vi "Prueba 2 Tania.vi"() -> ()   [LabVIEW 2013]
panel:
  out "mayor":dbl
  out "Menor":dbl
  out "Temperatura80":dbl
  out "Promedio":dbl
  out "Velocidad":i32(knob) scale=0.0..220.0
  # "Necesitamos generar 10 velocidades. \nal final de las 10 pruebas presentar :\n-Promedio de las velocidades mayores a 120\n-Velocidad Mayor y menor \n-Cuantas veces la temperatura fue mayor a 80"
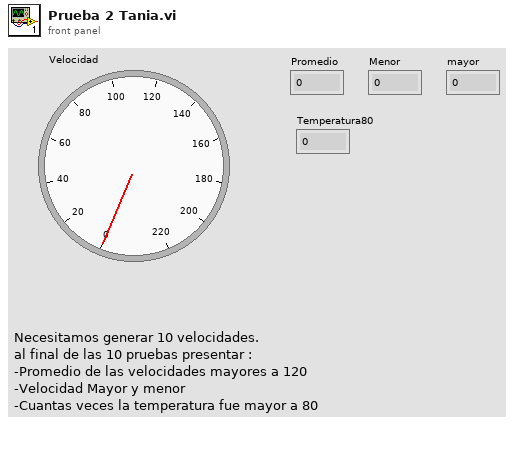
[diagram p1: front panel]
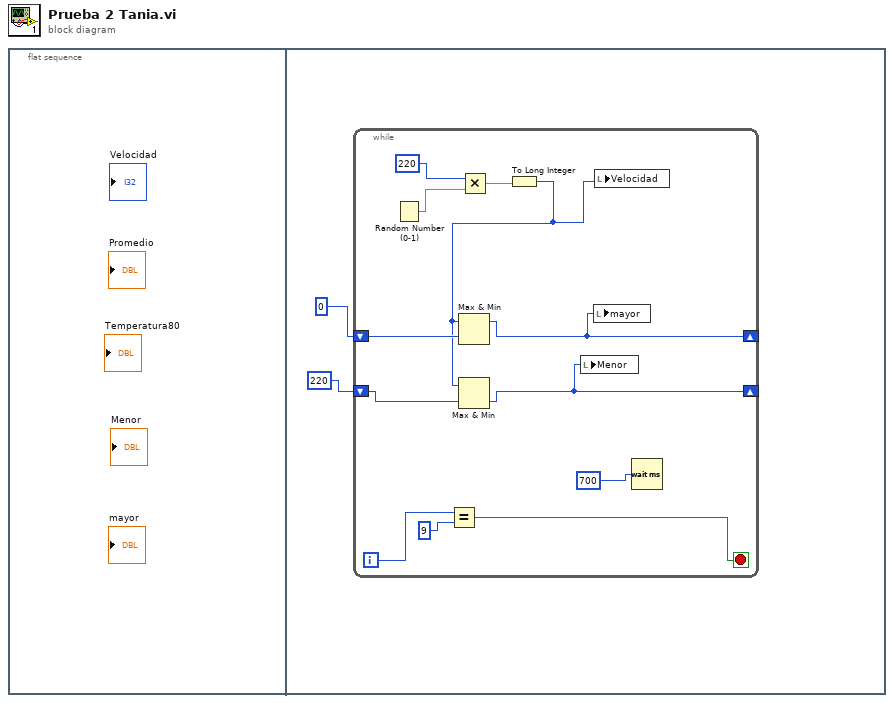
[diagram p0: block diagram]
diagram:
  n1 = flat-sequence {
    frame #0 {
    }
    frame #1 {
      n2 = while {
        shift-right: [w6] -> _
        shift-left: 0 -> [w7]
        shift-right: [w4] -> _
        shift-left: 220 -> [w5]
        i -> [w10]
        stop <- w9 stop-if-true
        n3 = Random Number (0-1)() -> (number: 0 to 1=w13:dbl)
        n4 = Equal?(x=w10, y=9) -> (x = y?=w9:bool)
        n5 = Multiply(x=220, y=w13) -> (x*y=w12:dbl)
        n6 = To Long Integer(number=w12) -> (32bit integer=w3:i32)
        n7 = Max & Min(x=w3, y=w7) -> (max(x,y)=w6:i32)  [unwired: 1 out]
        n8 = Max & Min(x=w3, y=w5) -> (min(x,y)=w4:i32)  [unwired: 1 out]
        n9 = local write "Menor"(w4) -> ()
        n10 = local write "mayor"(w6) -> ()
        n11 = local write "Velocidad"(w3) -> ()
        n12 = Wait (ms)(milliseconds to wait=700) -> ()  [unwired: 1 out]
      }
    }
  }
